vi "Stop Core.vi"(10 "final error code":i32, 11 "Tiff Writer in":refnum<class "Tiff Writer.lvclass">) -> (3 "Tiff Writer out":refnum<class "Tiff Writer.lvclass">)   [LabVIEW 2015, in "Tiff Writer.lvlib" / "Tiff Writer.lvclass"]
doc: "(<B>Filename</B>: Actor Framework.lvlib:Actor.lvclass:Stop Core.vi)\n\nDefines what the actor does before it stops. Use the <B>final error code</B> input to determine whether the actor shut down in response to an error.\n\nBy default, this method does nothing. A descendant class may override it to define behavior, such as shutting down any processes the actor initiated in its override of the Actor Core method."
uses:
  Tiff Writer.lvclass
  <vilib>/ActorFramework/Actor/Actor.lvclass
  BinaryTIFF/Classes/TIFF/TIFF.lvclass
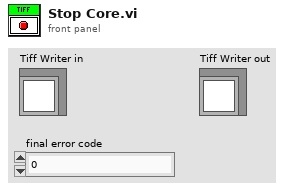
[diagram p1: front panel]
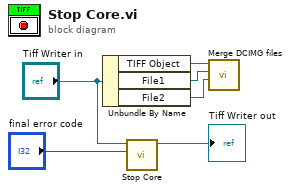
[diagram p0: block diagram]
diagram:
  n1 = Unbundle By Name("Tiff Writer in") -> ("TIFF Object"=w4:refnum<class "TIFF.lvclass">, "File1"=w3:path, "File2"=w2:path)
  n2 = call-parent "Stop Core.vi"("final error code"="final error code", "Actor in"="Tiff Writer in") -> ("Actor out"=→"Tiff Writer out":refnum<class "Tiff Writer.lvclass">)  [unwired: 9 in]
  n3 = call-dynamic "Merge DCIMG files.vi"("DCIMG Path 2"=w2, "DCIMG Path 1"=w3, "TIFF in"=w4) -> ()  [unwired: 7 in, 2 out]
